vi "log.vi"(0 "log string":string, 5 "logOption":string, 11 "error in (no error)":errorcluster) -> (15 "error out":errorcluster)   [LabVIEW 2017]
uses:
  <vilib>/NI VeriStand/Custom Device Tools/Custom Device Utility Library/Custom Device Utility Library.lvlib
  <vilib>/NI Veristand/Custom Device Tools/Custom Device Utility Library/RT Debug String Color Spec.ctl
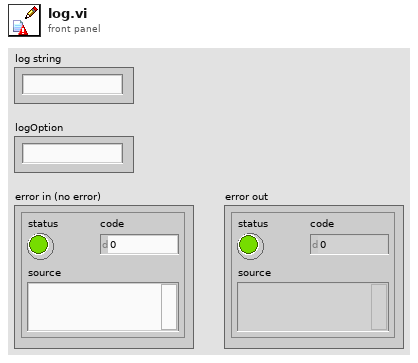
[diagram p1: front panel]
types:
  T1 = typedef "Custom Device Utility Library.lvlib/RT Debug String Color Spec.ctl" = u16
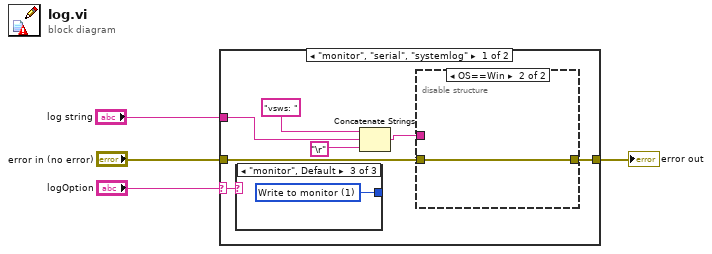
[diagram p0: block diagram]
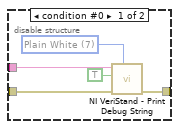
[diagram p2: hidden frame]
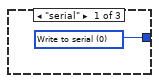
[diagram p3: hidden frame]
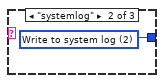
[diagram p4: hidden frame]
diagram:
  n1 = case shown="\"monitor\", \"serial\", \"systemlog\"" "logOption" {
    selector: "logOption" -> [w11 _]
    tunnel: "log string" -> [w9 _]
    tunnel: "error in (no error)" -> [w7 w21]
    tunnel: [w6 w21] -> w4
    frame "monitor", "serial", "systemlog" {
      n2 = case shown="\"monitor\", Default" w11 {
        tunnel: [w18 w19 w20] -> _
        frame "serial" {
          w18 = u16 0 items=["Write to serial", "Write to monitor", "Write to system log"] ("Interface")
        }
        frame "systemlog" {
          w19 = u16 2 items=["Write to serial", "Write to monitor", "Write to system log"] ("Interface")
        }
        frame "monitor", Default {
          w20 = u16 1 items=["Write to serial", "Write to monitor", "Write to system log"] ("Interface")
        }
      }
      n3 = Concatenate Strings("vsws: ", w9, "\r") -> (w5:string)
      n4 = disable-structure shown="OS==Win" {
        disable-tunnel: w7 -> [w15 w17]
        disable-tunnel: [w14 w17] -> w6
        disable-tunnel: w5 -> [w13 _]
        frame condition #0 {
          w16 = T1 7 items=["Plain White"=7, "Bold White"=15, "Bold Blue"=9, "Bold Green"=10, "Bold Red"=12] ("Attribute")
          n5 = call <vilib>:"NI VeriStand - Print Debug String.vi"("Attribute"=w16, "error in (no error)"=w15, "Add to log file? (T)"=TRUE, "Message"=w13) -> ("error out"=w14:errorcluster)  [unwired: 7 in]
        }
        frame condition #1 (active) {
        }
      }
    }
    frame "None", Default {
    }
  }
  "error out" <- w4
